vi "SystemNode_GetAttributes.vi"(0 "reference in":refnum<class "SystemNode.lvclass">, 5 "error in (no error)":errorcluster) -> (14 "reference out":refnum<class "SystemNode.lvclass">, 16 "Attributes":T1 {"Base class"."bounds"."height" format="%.2f"; "Base class"."bounds"."width" format="%.2f"; "Base class"."bounds"."y" format="%.2f"; "Base class"."bounds"."x" format="%.2f"}, 17 "Attributes locked?":bool, 19 "error out":errorcluster)   [LabVIEW 2012, in "SystemNode.lvclass"]
doc: "Returns the attributes of a SystemNode object.\n\nIf the object is currently locked for modification, 'Attributes locked?' will return TRUE.\n\n[GOOP 2.0.15]"
uses:
  <resource>/Framework/Providers/Open_GDS/UML/SystemNode_class/SystemNode.lvclass
  <resource>/Framework/Providers/Open_GDS/UML/SystemNode_class/protected/ObjectAttributes.ctl
  <resource>/Framework/Providers/Open_GDS/UML/AbstractNode_class/AbstractNode.lvclass
  <resource>/Framework/Providers/Open_GDS/UML/MultiLineString_class/MultiLineString.lvclass
  <resource>/Framework/Providers/Open_GDS/UML/RectangularNode_class/protected/ObjectAttributes.ctl
  <resource>/Framework/Providers/Open_GDS/UML/AbstractNode_class/protected/ObjectAttributes.ctl
  <resource>/Framework/Providers/Open_GDS/UML/General/Rectangle/Rectangle Rectangle2D.ctl
  <vilib>/addons/_goop3.llb/3GOOPStates.ctl
  <resource>/Framework/Providers/Open_GDS/UML/SystemNode_class/SystemNode.lvclass/SystemNode.ctl
  <resource>/Framework/Providers/Open_GDS/UML/RectangularNode_class/RectangularNode.lvclass
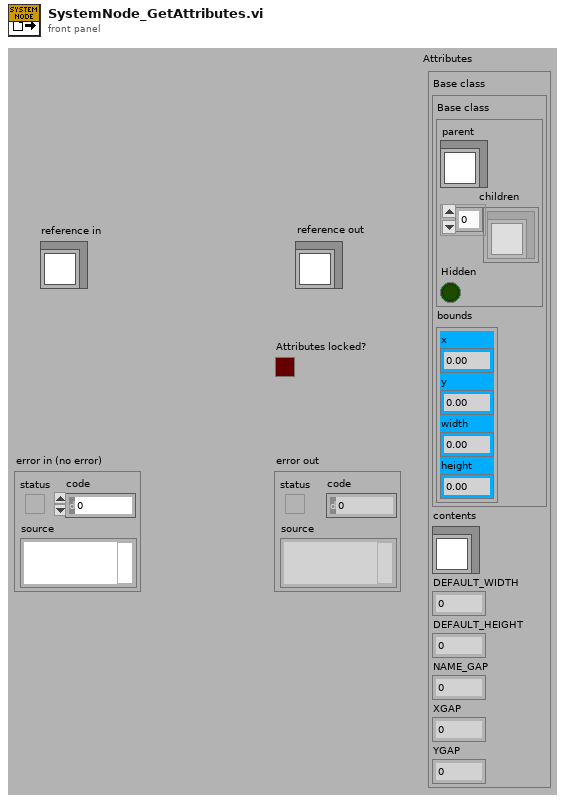
[diagram p1: front panel]
types:
  T1 = typedef "SystemNode.lvclass/ObjectAttributes.ctl" = cluster{"Base class":T2, "contents":refnum<class "MultiLineString.lvclass">, "DEFAULT_WIDTH":i32, "DEFAULT_HEIGHT":i32, "NAME_GAP":i32, "XGAP":i32, "YGAP":i32}
  T2 = typedef "RectangularNode.lvclass/ObjectAttributes.ctl" = cluster{"Base class":T3, "bounds":T4}
  T3 = typedef "AbstractNode.lvclass/ObjectAttributes.ctl" = cluster{"parent":refnum<class "AbstractNode.lvclass">, "children":refnum<class "AbstractNode.lvclass">[], "Hidden":bool}
  T4 = typedef "Rectangle Rectangle2D.ctl" = cluster{"x":dbl, "y":dbl, "width":dbl, "height":dbl}
  T5 = typedef "3GOOPStates.ctl" = enum16{"Set", "Get", "New", "Delete", "Clear", "Test and get", "Unlock data", "Information", "Look up existing", "New or look up existing", "Test and get shared", "Get shared", "Set shared", "Unlock shared", "Find dynamic method", "Register dynamic method", "Preload dynamic method", "Probe", "Cast to more generic", "Cast to more specific"}
  T6 = typedef "AbstractNode.lvclass/ObjectReference.ctl" = refnum<k1>
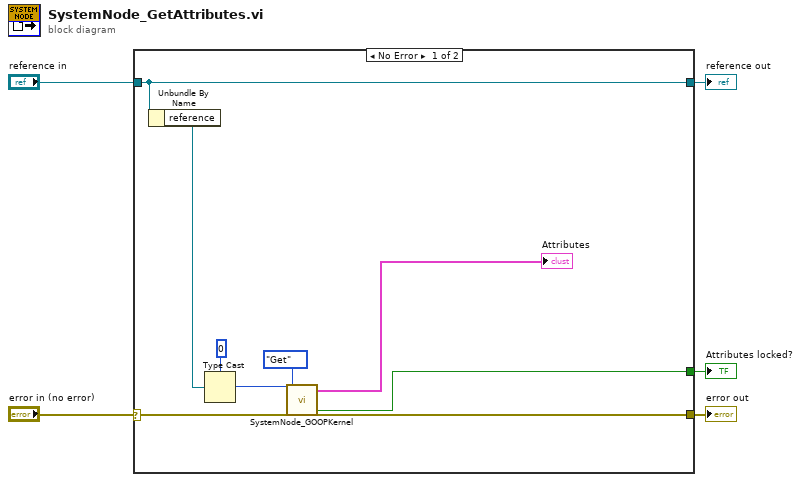
[diagram p0: block diagram]
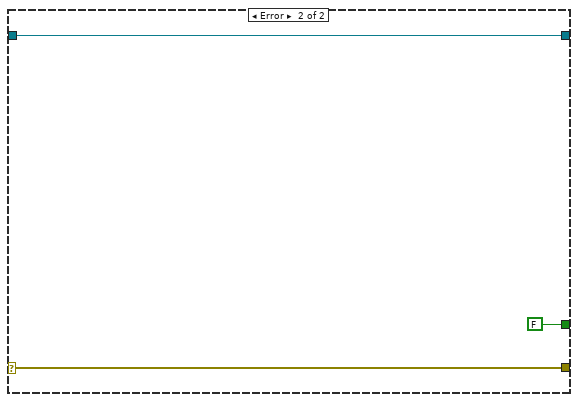
[diagram p2: hidden frame]
diagram:
  n1 = case shown="No Error" "error in (no error)" {
    selector: "error in (no error)" -> [w13 w16]
    tunnel: [w7 w17] -> w5
    tunnel: [w11 w16] -> w4
    tunnel: "reference in" -> [w7 w17]
    tunnel: [w10 FALSE ("Data locked?")] -> w1
    frame No Error {
      n2 = Unbundle By Name(w7) -> ("reference"=w6:T6)
      n3 = Type Cast(type=0, x=w6) -> (*(type *) &x=w12:i32)
      n4 = call <resource>:"SystemNode_GOOPKernel.vi"("Ref in"=w12, "error in (no error)"=w13, "Action"=3GOOPStates."Get") -> ("Data out"=→"Attributes":T1, "Data locked?"=w10:bool, "error out"=w11:errorcluster)  [unwired: 12 in, 10 out]
    }
    frame Error {
    }
  }
  "error out" <- w4
  "reference out" <- w5
  "Attributes locked?" <- w1
